vi "Write Multicolumn Listbox Headers (UTF-8 String).vi"(8 "error in":errorcluster, 9 "Row Headers":refnum<class "UTF-8 String.lvclass">[](array[class]), 10 "Column Headers":refnum<class "UTF-8 String.lvclass">[](array[class]), 11 "Control Ref":refnum<vi>) -> (0 "error out":errorcluster)   [LabVIEW 2020, in "G-Unicode.lvlib"]
doc: "Write and display unicode text in the headers of a multicolumn listbox control."
uses:
  G-Unicode.lvlib
  Types/UTF-8 String/UTF-8 String.lvclass
  Types/UTF-8 String/UTF-8 String.lvclass/UTF-8 String.ctl
  5206cb6b-04fb-41f5-a37e-29c14f142303.vi
  ac01c1c3-6448-4046-bb74-48d1977bc508.vi
  Private/Conversion/Text as Encoded String.vi
  Private/Conversion/Polymorphic VIs/Text as Encoded String (UTF-8 String).vi
  Private/Conversion/Encoded UTF-8 String to Encoded UTF-16LE String.vi
  Types/UTF-8 String/Read Encoded UTF-8 String.vi
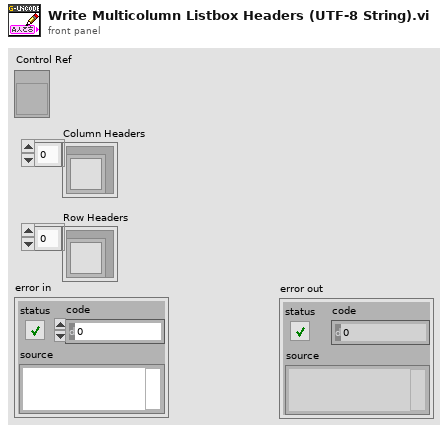
[diagram p1: front panel]
types:
  T1 = typedef "G-Unicode.lvlib/Encoded UTF-16LE String.ctl" = string
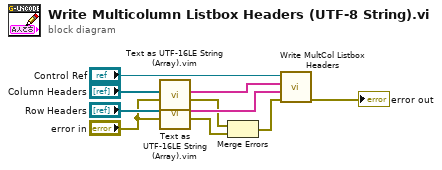
[diagram p0: block diagram]
diagram:
  n1 = call "Text as UTF-16LE String (Array).vim"("error in"="error in", "Text"="Column Headers") -> ("error out"=w3:errorcluster, "Encoded String"=w7:T1[])  [unwired: 8 in]
  n2 = call "Text as UTF-16LE String (Array).vim"("error in"="error in", "Text"="Row Headers") -> ("error out"=w2:errorcluster, "Encoded String"=w5:T1[])  [unwired: 8 in]
  n3 = Merge Errors(w3, w2) -> (w1:errorcluster)
  n4 = call "Write MultCol Listbox Headers.vi"("error in"=w1, "Row Headers"=w5, "Column Headers"=w7, "Multicolumn Listbox Ref in"="Control Ref") -> ("error out"=→"error out":errorcluster)  [unwired: 6 in, 1 out]
